vi "get_errorInfo.vi"(0 "HGF_Device_ErrorQuery":refnum<class "HGF_Device_ErrorQuery.lvclass">, 5 "error in (no error)":errorcluster) -> (14 "dup HGF_Device_ErrorQuery":refnum<class "HGF_Device_ErrorQuery.lvclass">, 15 "status":bool, 16 "errorCodes":i32[](array[numeric]), 17 "errorMessage":string, 19 "error out":errorcluster)   [LabVIEW 2014, in "HGF_DeviceBaseClasses.lvlib" / "HGF_Device_ErrorQuery.lvclass"]
doc: "This VI returns the result of the IDN query."
uses:
  HGF_Device_ErrorQuery.lvclass
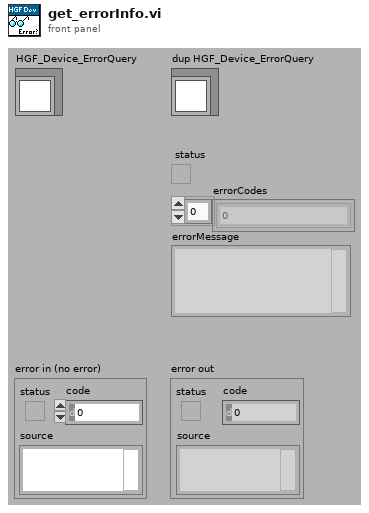
[diagram p1: front panel]
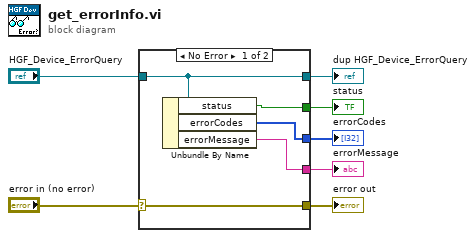
[diagram p0: block diagram]
diagram:
  n1 = case shown="No Error" "error in (no error)" {
    selector: "error in (no error)" -> [w12 w13]
    tunnel: [w12 w13] -> w6
    tunnel: [w11 w14] -> w4
    tunnel: "HGF_Device_ErrorQuery" -> [w11 w14]
    tunnel: [w10 _] -> w3
    tunnel: [w9 _] -> w2
    tunnel: [w8 _] -> w1
    frame No Error {
      n2 = Unbundle By Name(w11) -> ("status"=w10:bool, "errorCodes"=w9:i32[], "errorMessage"=w8:string)
    }
    frame Error {
    }
  }
  "error out" <- w6
  "dup HGF_Device_ErrorQuery" <- w4
  "errorMessage" <- w1
  "errorCodes" <- w2
  "status" <- w3
